vi "Configure and Start Housekeeping.vi"(8 "error in":errorcluster, 11 "PAS in":refnum<class "PAS.lvclass">) -> (0 "error out":errorcluster, 3 "PAS out":refnum<class "PAS.lvclass">)   [LabVIEW 2014, in "PAS.lvclass"]
doc: "VI for configuring and starting the housekeeping task. This VI defaults strictly to placing a housekeeping task named PAS Housekeeping into the class and starting the task."
uses:
  PAS.lvclass
  PAS.lvclass/PAS.ctl
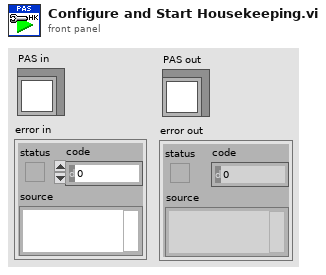
[diagram p1: front panel]
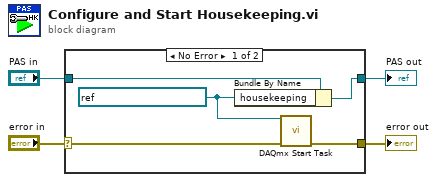
[diagram p0: block diagram]
diagram:
  n1 = case shown="No Error" "error in" {
    selector: "error in" -> [w9 w11]
    tunnel: [w8 w11] -> w3
    tunnel: [w6 w10] -> w1
    tunnel: "PAS in" -> [w7 w10]
    frame No Error {
      w5 = refnum<k21> "PAS Housekeeping" ("DAQmxTasks.housekeeping")
      n2 = Bundle By Name(cluster=w7, "housekeeping"=w5) -> (w6:refnum<class "PAS.lvclass">)
      n3 = call <vilib>:"DAQmx Start Task.vi"("task/channels in"=w5, "error in"=w9) -> ("error out"=w8:errorcluster)  [unwired: 12 in, 1 out]
    }
    frame Error {
    }
  }
  "error out" <- w3
  "PAS out" <- w1
